vi "Open_Next_File.vi"(5 "Input File Pattern":string="Test", 6 "Dir Path":path) -> (0 "Error Code":i32, 1 "Final File path":path, 2 "File Ref Num":refnum<file>, 3 "Output File Name":string, 4 "Stop":bool)   [LabVIEW 2019]
doc: "This VI takes a file name and keeps incrementing a tail until it can open a file that does not already exist. Scott Hannahs, FBNML, Jan 1992"
panel:
  out "Error Message":string
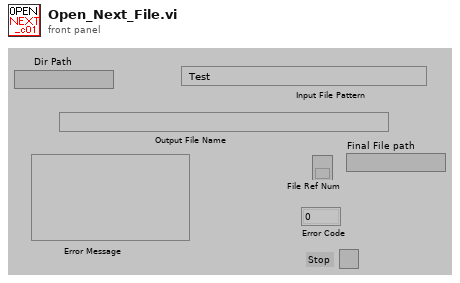
[diagram p1: front panel]
types:
  T1 = enum16{"open", "replace", "create", "open or create", "replace or create", "replace or create with confirmation"}
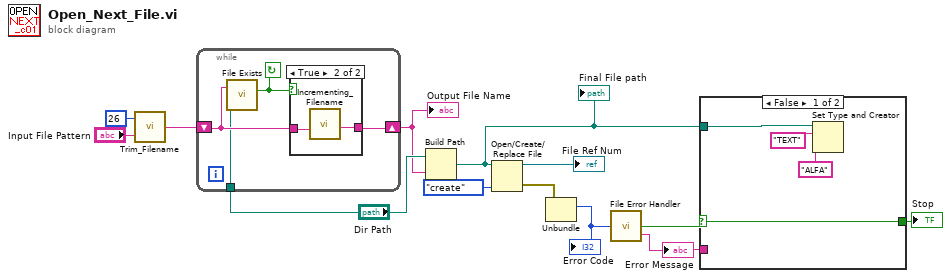
[diagram p0: block diagram]
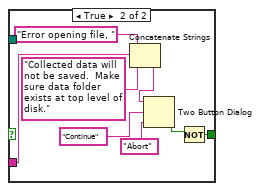
[diagram p3: hidden frame]
diagram:
  n1 = call "Trim_Filename.vi"("Input string"="Input File Pattern", "length"=26) -> ("output string"=w3:string)
  n2 = while {
    tunnel: "Dir Path" -> [w14]
    shift-left: w3 -> [w15]
    shift-right: [w16] -> w9
    stop <- w17 continue-if-true
    n3 = call "File Exists.vi"("Dir Path"=w14, "FILESPEC"=w15) -> (0:w17:bool)
    n4 = case shown="True" w17 {
      tunnel: w15 -> [w18 w19]
      tunnel: [w18 w20] -> w16
      frame False {
      }
      frame True {
        n5 = call "Incrementing_Filename.vi"("FILENAME IN"=w19) -> ("FILENAME OUT"=w20:string)
      }
    }
  }
  "Output File Name" <- w9
  n6 = Build Path(base path="Dir Path", name or relative path=w9) -> (appended path=w6:path)
  "Final File path" <- w6
  n7 = Open/Create/Replace File(file path (use dialog)=w6, operation (0:open)=T1."create") -> (refnum out=→"File Ref Num":refnum<file>, error out=w11:errorcluster)  [unwired: 4 in, 1 out]
  n8 = Unbundle(w11) -> ("code"=w4:i32)  [unwired: 2 out]
  "Error Code" <- w4
  n9 = call "File Error Handler.vi"("FILE SYSTEM\nERROR CODE"=w4) -> ("ERROR INDICATOR\nLED"=w13:bool, "ERROR MESSAGE"=w12:string)
  "Error Message" <- w12
  n10 = case shown="False" w13 {
    selector: w13 -> [w21 _]
    tunnel: w6 -> [w24 _]
    tunnel: [w21 w29] -> w5
    tunnel: w12 -> [_ w28]
    frame False {
      n11 = Set Type and Creator(5:"ALFA", 6:"TEXT", 7:w24) -> ()  [unwired: 1 in, 2 out]
    }
    frame True {
      n12 = Concatenate Strings("Error opening file, ", w28, "Collected data will not be saved.  Make sure data folder exists at top level of disk.") -> (w25:string)
      n13 = Two Button Dialog(message=w25, 1:"Abort", 2:"Continue") -> (T button?=w31:bool)
      n14 = Not(x=w31) -> (.not. x?=w29:bool)
    }
  }
  "Stop" <- w5
